vi "File Transfer DEBUG (RT).vi"() -> ()   [LabVIEW 2019]
uses:
  <vilib>/WebDAVClient/NI_WebDAV.lvlib
  <vilib>/WebDAVClient/Advanced/Put File.vi
panel:
  in  "Filename":string
  in  "Date":string
  in  "CA Number":string
  out "Time Elapsed (s)":dbl
  in  "Transfer":bool
  out "Array":string[](array[string])
  out "Waveform Chart":dbl(graph)
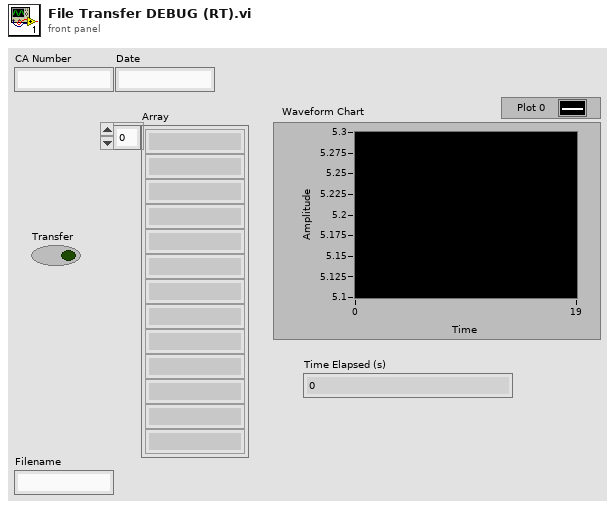
[diagram p1: front panel]
types:
  T1 = typedef "NI_WebDAV.lvlib/SessionHandle.ctl" = refnum<k1>
  T2 = typedef "NI_Real-Time Target Support.lvlib/RT CPU Load.ctl" = cluster{"Total (%)":dbl, "Time Critical (%)":dbl, "Timed Structures (%)":dbl, "High (%)":dbl, "Above Normal (%)":dbl, "Normal (%)":dbl, "Background (%)":dbl, "Idle (%)":dbl, "ISR (%)":dbl}
  T3 = enum16{"open", "replace", "create", "open or create", "replace or create", "replace or create with confirmation"}
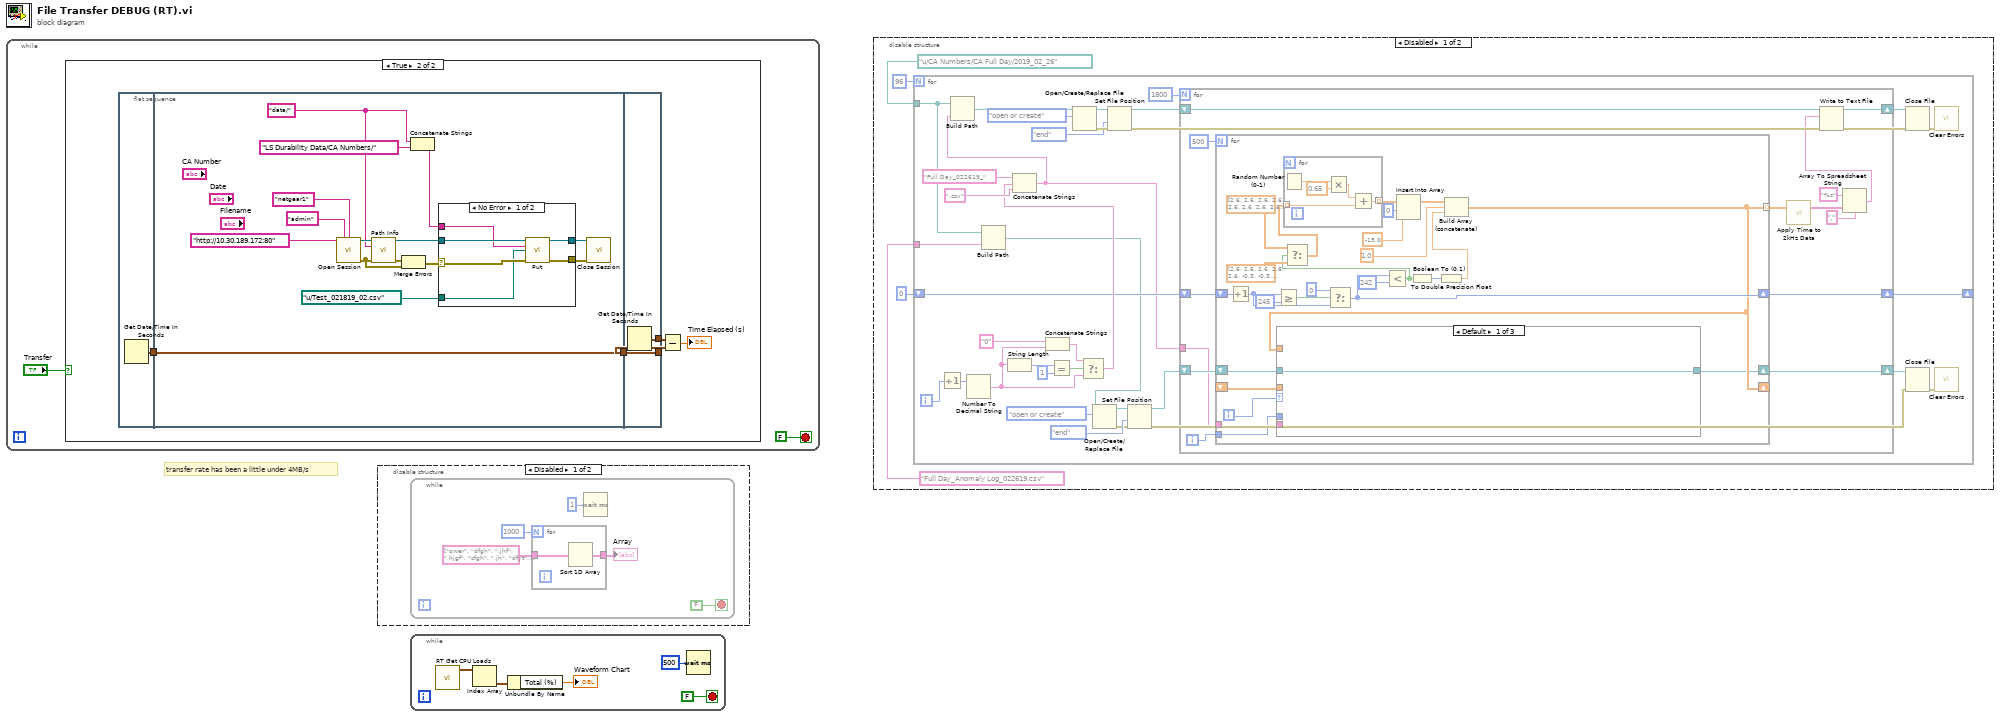
[diagram p0: block diagram]
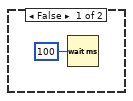
[diagram p2: hidden frame]
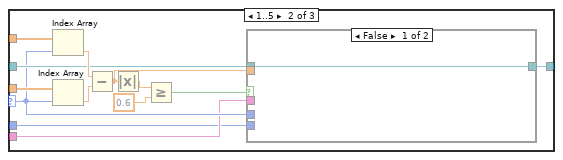
[diagram p4: hidden frame]
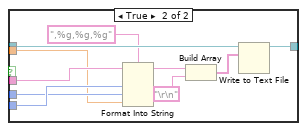
[diagram p5: hidden frame]
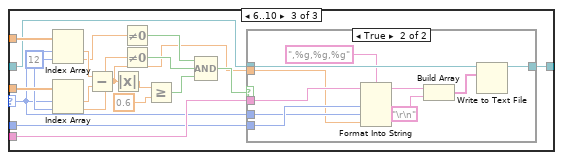
[diagram p6: hidden frame]
diagram:
  # "transfer rate has been a little under 4MB/s"
  n1 = while {
    stop <- FALSE stop-if-true
    n2 = case shown="True" "Transfer" {
      frame False {
        n3 = Wait (ms)(milliseconds to wait=u32 100) -> ()  [unwired: 1 out]
      }
      frame True {
        n4 = flat-sequence {
          tunnel: [w9] -> w7
          tunnel: w7 -> [w24]
          tunnel: [w24] -> w5
          tunnel: [w34] -> w8
          tunnel: [w33] -> w6
          tunnel: w5 -> [w33]
          frame #0 {
            n5 = Get Date/Time In Seconds() -> (seconds since 1Jan1904=w9:timestamp)
          }
          frame #1 {
            w11 = "data/" ("relative uri")
            n6 = call <vilib>:"Open Session.vi"("host uri prefix"="http://10.30.189.172:80", "username"="admin", "password"="netgear1") -> ("session handle out"=w18:T1, "error out"=w20:errorcluster)  [unwired: 11 in]
            n7 = call <vilib>:"Path Info.vi"("session handle"=w18, "relative uri"=w11, "error in (no error)"=w20) -> ("session handle out"=w17:T1, "error out"=w19:errorcluster)  [unwired: 9 in, 2 out]
            n8 = Merge Errors(w19, w20) -> (w15:errorcluster)
            n9 = Concatenate Strings(w11, "LS Durability Data/CA Numbers/" ("relative uri")) -> (w10:string)
            n10 = case shown="No Error" w15 {
              selector: w15 -> [w28 w32]
              tunnel: w17 -> [w30 w31]
              tunnel: [w29 w31] -> w16
              tunnel: [w27 w32] -> w14
              tunnel: path "u:/Test_021819_02.csv" -> [w26 _]
              tunnel: w10 -> [w25 _]
              frame No Error {
                n11 = call-poly <vilib>:"Put.vi"("session handle"=w30, "relative uri"=w25, "local file path"=w26, "error in (no error)"=w28) -> ("session handle out"=w29:T1, "error out"=w27:errorcluster)  [unwired: 9 in, 1 out]
              }
              frame Error {
              }
            }
            n12 = call <vilib>:"Close Session.vi"("session handle"=w16, "error in (no error)"=w14) -> ()  [unwired: 13 in, 1 out]
          }
          frame #2 {
            n13 = Get Date/Time In Seconds() -> (seconds since 1Jan1904=w34:timestamp)
          }
        }
        n14 = Subtract(x=w8, y=w6) -> (x-y=→"Time Elapsed (s)":dbl)
      }
    }
  }
  n15 = disable-structure shown="Disabled" {
    frame Disabled {
      n16 = while {
        stop <- FALSE stop-if-true
        n17 = for {
          N: 1000 -> [_]
          tunnel: string[] ["qwer", "dfgh", ",jhf", ",hjgf", "cfgh", ",jh", "dfyt", "jyhd", "iuytd", "yterw"] -> [w41]
          tunnel: [w40] -> w35
          n18 = Sort 1D Array(array=w41) -> (sorted array=w40:string[])
        }
        "Array" <- w35
        n19 = Wait (ms)(milliseconds to wait=u32 1) -> ()  [unwired: 1 out]
      }
    }
    frame Enabled {
    }
  }
  n20 = while {
    stop <- FALSE stop-if-true
    n21 = call <vilib>:"RT Get CPU Loads.vi"() -> ("CPU loads"=w46:T2[])  [unwired: 10 in, 1 out]
    n22 = Index Array(array=w46) -> (element=w45:T2)  [unwired: 1 in]
    n23 = Unbundle By Name(w45) -> ("Total (%)"=→"Waveform Chart":dbl)
    n24 = Wait (ms)(milliseconds to wait=u32 500) -> ()  [unwired: 1 out]
  }
  n25 = disable-structure shown="Disabled" {
    frame Disabled {
      n26 = for {
        N: 96 -> [_]
        tunnel: path "u:/CA Numbers/CA Full Day/2019_02_26" -> [w62]
        shift-right: [w63] -> _
        shift-left: 0 -> [w64]
        tunnel: "Full Day_Anomaly Log_022619.csv" -> [w61]
        i -> [w83]
        n27 = Increment(x=w83) -> (x+1=w82:i32)
        n28 = Number To Decimal String(number=w82) -> (decimal integer string=w77:string)  [unwired: 1 in]
        n29 = Build Path(base path=w62, name or relative path=w61) -> (appended path=w55:path)
        n30 = String Length(string=w77) -> (length=w81:i32)
        n31 = Concatenate Strings("0", w77) -> (w76:string)
        n32 = Equal?(x=w81, y=1) -> (x = y?=w79:bool)
        n33 = Select(t=w76, s=w79, f=w77) -> (s? t:f=w75:string)
        n34 = Concatenate Strings("Full Day_022619_", w75, ".csv") -> (w60:string)
        n35 = Build Path(base path=w62, name or relative path=w60) -> (appended path=w68:path)
        n36 = Open/Create/Replace File(file path (use dialog)=w68, operation (0:open)=T3."open or create") -> (refnum out=w71:refnum<file>, error out=w70:errorcluster)  [unwired: 4 in, 1 out]
        n37 = Open/Create/Replace File(file path (use dialog)=w55, operation (0:open)=T3."open or create") -> (refnum out=w57:refnum<file>, error out=w58:errorcluster)  [unwired: 4 in, 1 out]
        n38 = Set File Position(refnum=w71, from (0:start)=enum16{"start", "end", "current"}."end", error in=w70) -> (refnum out=w67:refnum<file>, error out=w65:errorcluster)  [unwired: 1 in]
        n39 = Set File Position(refnum=w57, from (0:start)=enum16{"start", "end", "current"}."end", error in=w58) -> (refnum out=w54:refnum<file>, error out=w51:errorcluster)  [unwired: 1 in]
        n40 = for {
          N: 1800 -> [_]
          shift-right: [w97] -> w66
          shift-left: w67 -> [w98]
          shift-right: [w94] -> w63
          shift-left: w64 -> [w95]
          tunnel: w60 -> [w87]
          shift-right: [w92] -> w53
          shift-left: w54 -> [w93]
          i -> [w86]
          n41 = for {
            N: 500 -> [_]
            tunnel: [w104] -> w96 mode=indexing
            shift-right: [w114] -> w94
            shift-left: w95 -> [w120]
            shift-right: [w104] -> _
            shift-left: _ -> [w106]
            shift-right: [w102] -> w92
            shift-left: w93 -> [w103]
            tunnel: w87 -> [w101]
            tunnel: w86 -> [w100]
            i -> [w105]
            n42 = Increment(x=w120) -> (x+1=w117:i32)
            n43 = Greater Or Equal?(x=w117, y=245) -> (x >= y?=w119:bool)
            n44 = Select(t=0, s=w119, f=w117) -> (s? t:f=w114:i32)
            n45 = Less?(x=w114, y=242) -> (x < y?=w107:bool)
            n46 = Select(t=dbl[] [2.6, 2.6, 2.6, 2.6, 2.6, 2.6, 2.6, 2.6, 2.6, 2.6, 4.65], s=w107, f=dbl[] [2.6, 2.6, 2.6, 2.6, 2.6, -0.3, -0.3, -0.3, -0.3, -0.3, 4.65]) -> (s? t:f=w110:dbl[])
            n47 = for {
              tunnel: w110 -> [w181] mode=indexing
              tunnel: [w180] -> w124 mode=indexing
              n48 = Random Number (0-1)() -> (number: 0 to 1=w184:dbl)
              n49 = Multiply(x=w184, y=0.65) -> (x*y=w182:dbl)
              n50 = Add(x=w182, y=w181) -> (x+y=w180:dbl)
            }
            n51 = Insert Into Array(array=w124, index=0, new element=-15.0) -> (w121:dbl[])
            n52 = Boolean To (0,1)(Boolean=w107) -> (0, 1=w112:i16)
            n53 = To Double Precision Float(number=w112) -> (double precision float=w111:dbl)
            n54 = Build Array (concatenate)(w121, 1.0, w111) -> (w104:dbl[])
            n55 = case shown="Default" w105 {
              selector: w105 -> [_ w129 w150]
              tunnel: w106 -> [_ w138 w168]
              tunnel: w104 -> [_ w137 w167]
              tunnel: w103 -> [w125 w131 w153]
              tunnel: [w125 w130 w154] -> w102
              tunnel: w101 -> [_ w128 w155]
              tunnel: w100 -> [_ w127 w151]
              frame Default {
              }
              frame 1..5 {
                n56 = Index Array(array=w137, index=w129) -> (element=w136:dbl)
                n57 = Index Array(array=w138, index=w129) -> (element=w135:dbl)
                n58 = Subtract(x=w136, y=w135) -> (x-y=w126:dbl)
                n59 = Absolute Value(x=w126) -> (abs(x)=w134:dbl)
                n60 = Greater Or Equal?(x=w134, y=0.6) -> (x >= y?=w132:bool)
                n61 = case shown="False" w132 {
                  tunnel: w131 -> [w139 w149]
                  tunnel: [w139 w148] -> w130
                  tunnel: w129 -> [_ w144]
                  tunnel: w128 -> [_ w147]
                  tunnel: w127 -> [_ w145]
                  tunnel: w126 -> [_ w143]
                  frame False {
                  }
                  frame True {
                    n62 = Format Into String(format string=",%g,%g,%g", initial string=w147, w145, w144, w143) -> (resulting string=w142:string)  [unwired: 1 in, 1 out]
                    n63 = Build Array(w142, "\r\n") -> (w140:string[])
                    n64 = Write to Text File(file (use dialog)=w149, text=w140) -> (refnum out=w148:refnum<file>)  [unwired: 2 in, 2 out]
                  }
                }
              }
              frame 6..10 {
                w162 = 12 ("index")
                n65 = Index Array(array=w167, index #1=w150, index #2=w162) -> (element #1=w166:dbl, element #2=w161:dbl)
                n66 = Index Array(array=w168, index #1=w150, index #2=w162) -> (element #1=w165:dbl, element #2=w160:dbl)
                n67 = Subtract(x=w166, y=w165) -> (x-y=w152:dbl)
                n68 = Absolute Value(x=w152) -> (abs(x)=w164:dbl)
                n69 = Not Equal To 0?(x=w161) -> (x != 0?=w159:bool)
                n70 = Not Equal To 0?(x=w160) -> (x != 0?=w158:bool)
                n71 = Greater Or Equal?(x=w164, y=0.6) -> (x >= y?=w157:bool)
                n72 = Compound Arithmetic op=AND(w159, w158, w157) -> (w156:bool)
                n73 = case shown="True" w156 {
                  tunnel: w153 -> [w169 w179]
                  tunnel: [w169 w178] -> w154
                  tunnel: w150 -> [_ w174]
                  tunnel: w155 -> [_ w177]
                  tunnel: w151 -> [_ w175]
                  tunnel: w152 -> [_ w173]
                  frame False {
                  }
                  frame True {
                    n74 = Format Into String(format string=",%g,%g,%g", initial string=w177, w175, w174, w173) -> (resulting string=w172:string)  [unwired: 1 in, 1 out]
                    n75 = Build Array(w172, "\r\n") -> (w170:string[])
                    n76 = Write to Text File(file (use dialog)=w179, text=w170) -> (refnum out=w178:refnum<file>)  [unwired: 2 in, 2 out]
                  }
                }
              }
            }
          }
          n77 = call "Apply Time to 2kHz Data.vi"("Data In"=w96) -> ("Data Out"=w90:string[][])  [unwired: 2 in, 1 out]
          n78 = Array To Spreadsheet String(delimiter (Tab)=",", array=w90, 3:"%s" ("format string")) -> (spreadsheet string=w89:string)
          n79 = Write to Text File(file (use dialog)=w98, text=w89) -> (refnum out=w97:refnum<file>)  [unwired: 2 in, 2 out]
        }
        n80 = Close File(refnum=w66, error in=w65) -> (error out=w73:errorcluster)  [unwired: 1 out]
        n81 = Close File(refnum=w53, error in=w51) -> (error out=w52:errorcluster)  [unwired: 1 out]
        n82 = call <vilib>:"Clear Errors.vi"("error in (no error)"=w73) -> ()  [unwired: 5 in, 2 out]
        n83 = call <vilib>:"Clear Errors.vi"("error in (no error)"=w52) -> ()  [unwired: 5 in, 2 out]
      }
    }
    frame Enabled {
    }
  }
